vi "Destroy.vi"(8 "error in (no error)":errorcluster, 11 "obj":refnum<class "Bike.lvclass">) -> (0 "error out":errorcluster)   [LabVIEW 2019, in "Bike.lvclass"]
doc: "Destroys the by ref object.\n\nwww.sciware.com.au\nBSD License (http://www.opensource.org/licenses/bsd-license.php)"
uses:
  Bike.lvclass
  Bike.lvclass/Bike.ctl
panel:
  # "BSD License (http://www.opensource.org/licenses/bsd-license.php)"
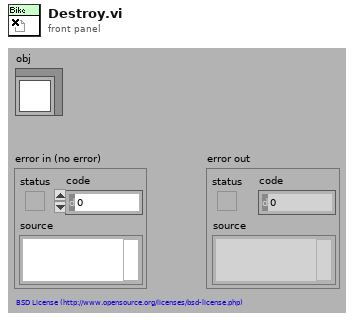
[diagram p1: front panel]
types:
  T1 = typedef "Bike.lvclass/DataRef.ctl" = refnum<data-value>
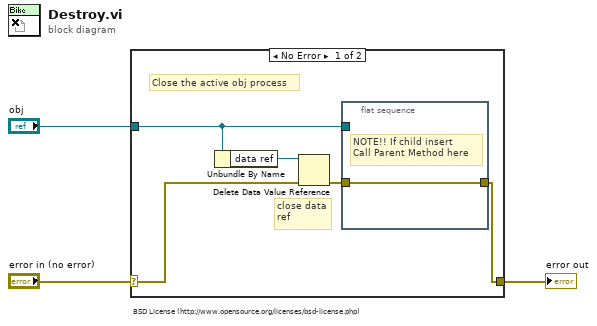
[diagram p0: block diagram]
diagram:
  # "BSD License (http://www.opensource.org/licenses/bsd-license.php)"
  n1 = case shown="No Error" "error in (no error)" {
    selector: "error in (no error)" -> [w4 w10]
    tunnel: [w6 w10] -> w2
    tunnel: "obj" -> [w5 _]
    frame No Error {
      # "close data\nref"
      # "Close the active obj process"
      n2 = Unbundle By Name(w5) -> ("data ref"=w8:T1)
      n3 = Delete Data Value Reference(data value reference=w8, error in=w4) -> (error out=w7:errorcluster)  [unwired: 1 out]
      n4 = flat-sequence {
        tunnel: w7 -> [w9]
        tunnel: [w9] -> w6
        tunnel: w5 -> [_]
        frame #0 {
          # "NOTE!! If child insert\nCall Parent Method here"
        }
      }
    }
    frame Error {
    }
  }
  "error out" <- w2
